vi "Tetra Serial.vi"(0 "COMPORT":refnum<visa-resource-name>="COM4", 1 "Delay Time (ms)":dbl=1.0 caption="Delay Time (s)", 7 "ClearErrorIn(t)":bool=TRUE, 9 "Timeout(s)":dbl=10.0 format="%#_13g", 11 "error in (no error)":errorcluster, 12 "Command":string, 13 "Open Ser(t)":bool, 14 "Close Ser(t)":bool) -> (2 "Success":bool=TRUE, 3 "output":string="adcframe\r\nADC0 Frame: 0x3000800600800655\r\nADC1 Frame: 0x31FF2FF2FF2FF214\r\nADC2 Frame: 0x32FF6FF6FF7FF651\r\nADC3 Frame: 0x33FF1FF0FF3FF033\r\n>", 4 "comport":refnum<visa-resource-name>="COM4", 8 "Timeout":bool caption="Time has Elapsed", 15 "error out":errorcluster)   [LabVIEW 2018]
doc: "This example performs writes and reads on a serial port, as directed by the user. You can press the Write and Read buttons, and change the Read Count, while the example is running.\n\nThe parameters set for the serial port must match the parameters of the connected instrument or device. In this example, the Read Count parameter specifies the number of bytes that the serial port reads. If there were more bytes at the port than the specified number, those bytes would not be read. If there were less bytes at the port than the specified number, you would receive a timeout error.\n\nThis example expands upon the flow control options for XON and XOFF, allowing the user to choose those control characters. Also, the user can enable or disable a termination character. Some devices require a termination character in order to identify the end of command strings. Some devices send a termination character to signify the end of data to be read. This example shows how you can end the Read operation once a termination character is detected in the buffer and/or append a termination character at the end of the Write data."
uses:
  Program Files (x86)/National Instruments/LabVIEW 2018/examples/Instrument IO/Serial/support/Serial - Settings.ctl
  Program Files (x86)/National Instruments/LabVIEW 2018/examples/Instrument IO/Serial/support/Serial - XON-XOFF Characters.ctl
  Program Files (x86)/National Instruments/LabVIEW 2018/examples/Instrument IO/Serial/support/Serial - ASCII Characters.ctl
  <vilib>/Instr/_visa.llb/VISA Flush IO Buffer Mask.ctl
  <vilib>/Utility/error.llb/DialogType.ctl
  Tetra_Globals.vi
  <vilib>/Instr/_visa.llb/VISA Configure Serial Port (Instr).vi
panel:
  out "before substring":string
  out "VI Name":string="Tetra Serial.vi"
  out "x > y?":bool
  in  "set size (in Mbytes)":i64=60
  out "size (in bytes)":i64=140690
  out "file or folder exists?":bool=TRUE
  out "NaN/Path/Refnum?":bool
  out "record id":string="02222023100252"
  in  "Tab Control":enum32{"Page 1", "Page 2"}(tab)
  in  "-ssid":string="123"
  out "Error":bool=TRUE
  out "Elapsed Time (s)":dbl=2.479999966453761e-05
  out "Time(s)":dbl=0.03430839999964519
  in  "x":bool
  in  "LogCapturestoFile":bool
  out "LogFilePath":string="C:\\RageATE Results\\Serial Logs\\02222023100252.txt"
  in  "Read Count":u32=1
  out "return count":u32=8
  out "Numeric Control":i32=138
  in  "Max Lines to Read":i32=1000
  in  "Serial Settings":T1={"baud rate"=115200, "data bits"=8, "parity"=enum."None", "stop bits"=10, "flow control"=0} {"flow control" items=["None"=0, "XON/XOFF"=1, "RTS/CTS"=2, "DTR/DSR"=4]; "stop bits" items=["1.0"=10, "1.5"=15, "2.0"=20]; "data bits" min=5 max=8 step=1; "baud rate" items=["75"=75, "110"=110, "134"=134, "150"=150, "300"=300, "600"=600, "1200"=1200, "1800"=1800, "2400"=2400, "4800"=4800, "7200"=7200, "9600"=9600, "14400"=14400, "19200"=19200, "28800"=28800, "38400"=38400, "56000"=56000, "57600"=57600, "115200"=115200, "128000"=128000, "230400"=230400]}
  in  "XON/XOFF Characters":T2={"XON"=enum."DC1", "XOFF"=enum."DC3"}
  in  "Termination Character":u8=10 format="%.0x"
  out "refnum out":refnum<file>
  out "Start(s)":dbl=8979.5775258 format="%_19f"
  out "log":string="id: 02222023100252 date: 22/02/23  12:18:52.6692  OpenSer: FALSE CloseSer: FALSE  success: TRUE  timeout: FALSE  comport: COM4  cmd: adcframe  return: adcframe;ADC0 Frame: 0x3000800600800655;ADC1 Frame: 0x31FF2FF2FF2FF214;ADC2 Frame: 0x32FF6FF6FF7FF651;ADC3 Frame: 0x33FF1FF0FF3FF033;>"
  # "0xA is equivalent to a '\\n' character, which is a line feed."
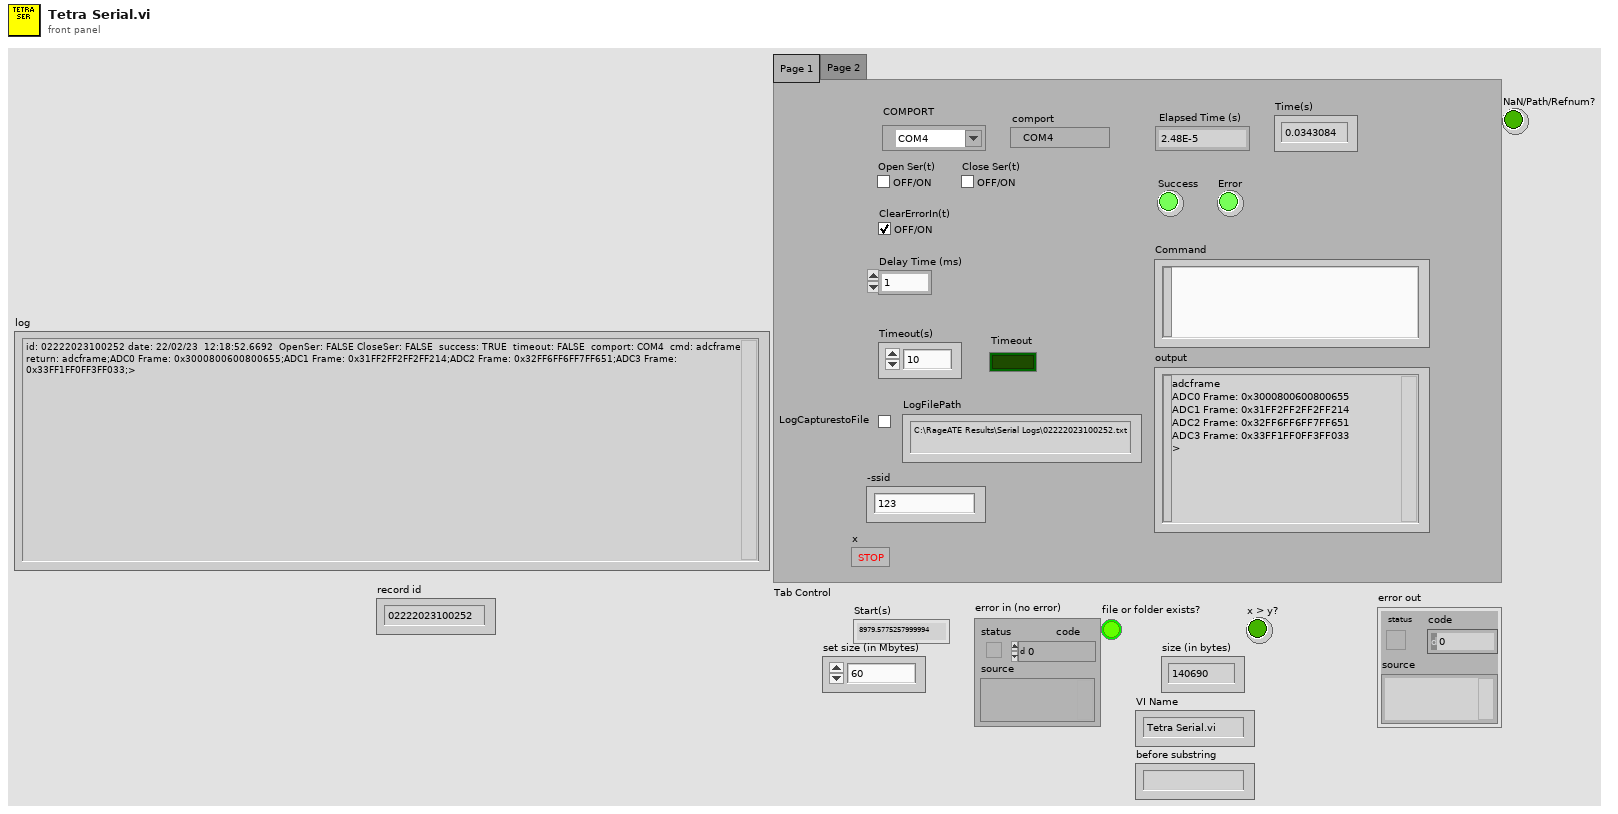
[diagram p1: front panel]
types:
  T1 = typedef "Serial - Settings.ctl" = cluster{"baud rate":u32, "data bits":u16, "parity":enum16{"None", "Odd", "Even", "Mark", "Space"}, "stop bits":u16, "flow control":u16}
  T2 = typedef "Serial - XON-XOFF Characters.ctl" = cluster{"XON":T3, "XOFF":T3}
  T3 = typedef "Serial - ASCII Characters.ctl" = enum16{"NUL", "SOH", "STX", "ETX", "EOT", "ENQ", "ACK", "BEL", "BS", "HT", "LF", "VT", "FF", "CR", "SO", "SI", "DLE", "DC1", "DC2", "DC3", "DC4", "NAK", "SYN", "ETB", "CAN", "EM", "SUB", "ESC", "FS", "GS", "RS", "US", "SP", "!", "\"", "#", "$", "%", "&", "'", "(", ")", "*", "+", ",", "- (-)", ".", "/", "0", "1", "2", "3", "4", "5", "6", "7", "8", "9", ":", ";", "<", "=", ">", "?", "@", "A", "B", "C", "D", "E", "F", "G", "H", "I", "J", "K", "L", "M", "N", "O", "P", "Q", "R", "S", "T", "U", "V", "W", "X", "Y", "Z", "[", "\\", "]", "^", "_", "`", "a", "b", "c", "d", "e", "f", "g", "h", "i", "j", "k", "l", "m", "n", "o", "p", "q", "r", "s", "t", "u", "v", "w", "x", "y", "z", "{", "|", "}", "~"}
  T4 = enum16{"open", "replace", "create", "open or create", "replace or create", "replace or create with confirmation"}
  T5 = typedef "VISA Flush IO Buffer Mask.ctl" = u16
  T6 = typedef "DialogType.ctl" = u16
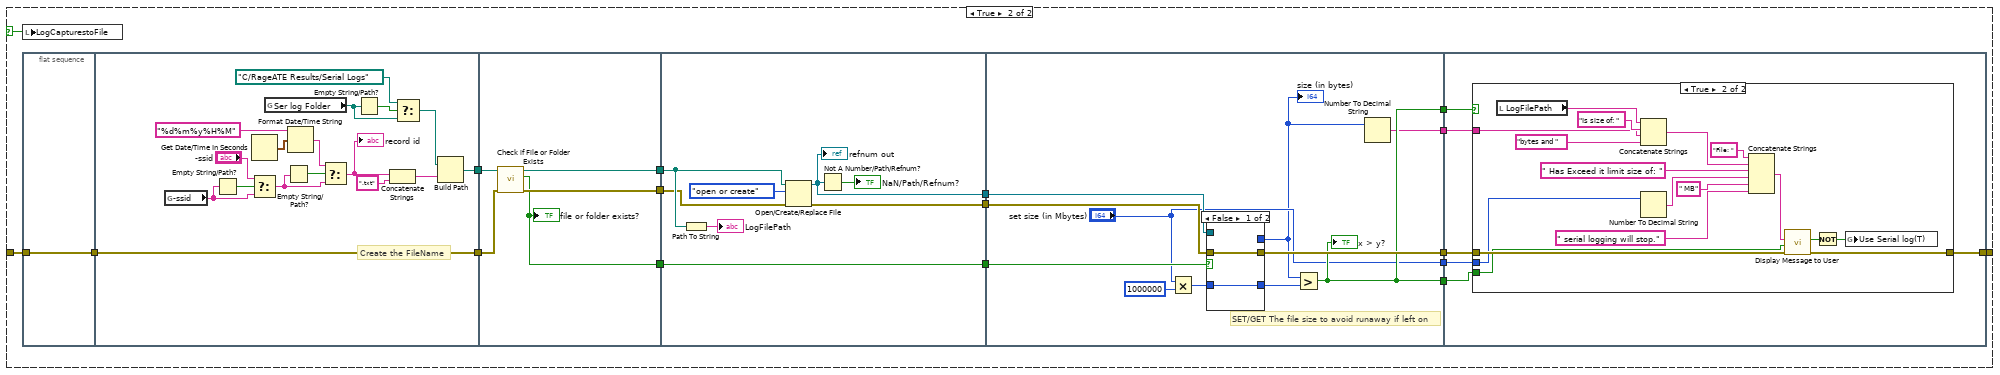
[diagram p2: hidden frame]
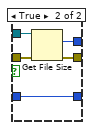
[diagram p3: hidden frame]
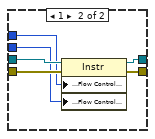
[diagram p8: hidden frame]
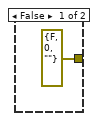
[diagram p9: hidden frame]
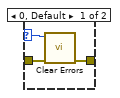
[diagram p10: hidden frame]
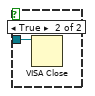
[diagram p12: hidden frame]
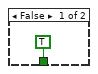
[diagram p14: hidden frame]
diagram:
  n1 = for {
    N: 1 -> [_]
    tunnel: [w5] -> w2
    stop <- w3 stop-if-true
    n2 = flat-sequence {
      tunnel: ["COMPORT"] -> w13
      tunnel: [w17] -> w12
      tunnel: [w118] -> w9
      tunnel: [w117] -> w10
      tunnel: w13 -> [w120]
      tunnel: w12 -> [w119]
      tunnel: [w115] -> w11
      tunnel: [w356] -> w8
      tunnel: [w355] -> w7
      tunnel: w11 -> [w353]
      tunnel: w10 -> [w356]
      tunnel: w9 -> [w355]
      tunnel: [w353] -> w6
      tunnel: w8 -> [_]
      tunnel: w7 -> [w359]
      tunnel: w6 -> [w360]
      tunnel: [w358] -> w4
      tunnel: [w386] -> w5
      tunnel: w4 -> [w386]
      tunnel: [w384] -> w3
      frame #0 {
        n3 = property class="VI"() -> ("Name"=→"VI Name":string)  [unwired: 2 in, 2 out]
        n4 = call <vilib>:"High Resolution Relative Seconds.vi"() -> ("relative seconds"=→"Start(s)":dbl)
        n5 = local write "output"("") -> ()
        n6 = global read "Tetra_Globals.vi" "Use Serial log(T)"() -> (w19:bool)
        n7 = local write "x"(FALSE ("x")) -> ()
        n8 = Or(x="LogCapturestoFile", y=w19) -> (x .or. y?=w20:bool)
        n9 = case shown="False" w20 {
          selector: w20 -> [_ w41]
          tunnel: "error in (no error)" -> [w24 w37]
          tunnel: [w24 w29] -> w17
          frame False {
          }
          frame True {
            n10 = local write "LogCapturestoFile"(w41) -> ()
            n11 = flat-sequence {
              tunnel: w37 -> [w42]
              tunnel: [w42] -> w26
              tunnel: [w45] -> w40
              tunnel: [w43] -> w36
              tunnel: w26 -> [w43]
              tunnel: w40 -> [w62]
              tunnel: [w64] -> w39
              tunnel: [w63] -> w38
              tunnel: w36 -> [w61]
              tunnel: [w60] -> w33
              tunnel: w39 -> [w69]
              tunnel: w38 -> [w70]
              tunnel: [w67] -> w35
              tunnel: [w66] -> w34
              tunnel: w33 -> [w65]
              tunnel: [w65] -> w32
              tunnel: w35 -> [w83]
              tunnel: w34 -> [w82]
              tunnel: w32 -> [w81]
              tunnel: ["set size (in Mbytes)"] -> w31
              tunnel: [w80] -> w30
              tunnel: [w79] -> w28
              tunnel: [w79] -> w27
              tunnel: [w74] -> w25
              tunnel: w31 -> [w94]
              tunnel: w30 -> [w96]
              tunnel: [w95] -> w29
              tunnel: w28 -> [w93]
              tunnel: w27 -> [w92]
              tunnel: w25 -> [w91]
              frame #0 {
              }
              frame #1 {
                # "Create the FileName"
                n12 = global read "Tetra_Globals.vi" "-ssid"() -> (w51:string)
                n13 = Empty String/Path?(string/path=w51) -> (empty?=w52:bool)
                n14 = Get Date/Time In Seconds() -> (seconds since 1Jan1904=w58:timestamp)
                n15 = Select(t="-ssid", s=w52, f=w51) -> (s? t:f=w49:string)
                n16 = global read "Tetra_Globals.vi" "Ser log Folder"() -> (w48:path)
                n17 = Empty String/Path?(string/path=w49) -> (empty?=w59:bool)
                n18 = Format Date/Time String(time format string (%c)="%d%m%y%H%M", seconds (now)=w58) -> (date/time string=w56:string)  [unwired: 1 in]
                n19 = Select(t=w56, s=w59, f=w49) -> (s? t:f=w55:string)
                "record id" <- w55
                n20 = Empty String/Path?(string/path=w48) -> (empty?=w47:bool)
                n21 = Concatenate Strings(w55, ".txt" ("string")) -> (w53:string)
                n22 = Select(t=path "C:/RageATE Results/Serial Logs" ("base path"), s=w47, f=w48) -> (s? t:f=w44:path)
                n23 = Build Path(base path=w44, name or relative path=w53) -> (appended path=w45:path)
              }
              frame #2 {
                n24 = call <vilib>:"Check if File or Folder Exists.vi"("error in (no error)"=w61, "path"=w62) -> ("error out"=w64:errorcluster, "file or folder exists?"=w60:bool, "dup path"=w63:path)  [unwired: 7 in]
                "file or folder exists?" <- w60
              }
              frame #3 {
                n25 = Path To String(path=w70) -> (string=→"LogFilePath":string)
                n26 = Open/Create/Replace File(file path (use dialog)=w70, error in=w69, operation (0:open)=T4."open or create") -> (refnum out=w66:refnum<file>, error out=w67:errorcluster)  [unwired: 3 in, 1 out]
                "refnum out" <- w66
                n27 = Not A Number/Path/Refnum?(number/path/refnum=w66) -> (NaN/Path/Refnum?=→"NaN/Path/Refnum?":bool)
              }
              frame #4 {
                # "SET/GET The file size to avoid runaway if left on"
                n28 = Multiply(x="set size (in Mbytes)", y=i64 1000000) -> (x*y=w76:i64)
                n29 = case shown="False" w81 {
                  tunnel: w83 -> [w84 w89]
                  tunnel: w82 -> [_ w90]
                  tunnel: [_ w86] -> w75
                  tunnel: w76 -> [w85 w87]
                  tunnel: [w84 w88] -> w80
                  tunnel: [w85 w87] -> w73
                  frame False {
                  }
                  frame True {
                    n30 = Get File Size(file=w90, error in=w89) -> (size (in bytes)=w86:i64, 0:w88:errorcluster)  [unwired: 1 out]
                  }
                }
                "size (in bytes)" <- w75
                n31 = Greater?(x=w75, y=w73) -> (0:w79:bool)
                "x > y?" <- w79
                n32 = Number To Decimal String(number=w75) -> (decimal integer string=w74:string)  [unwired: 1 in]
              }
              frame #5 {
                n33 = case shown="True" w92 {
                  tunnel: w96 -> [w97 w114]
                  tunnel: [w97 w113] -> w95
                  tunnel: w94 -> [_ w109]
                  tunnel: w93 -> [_ w105]
                  tunnel: w91 -> [_ w99]
                  frame False {
                  }
                  frame True {
                    n34 = local read "LogFilePath"() -> (w111:string)
                    n35 = Concatenate Strings(w111, "Is size of: " ("string"), w99, "bytes and " ("string")) -> (w101:string)
                    n36 = Number To Decimal String(number=w109) -> (decimal integer string=w108:string)  [unwired: 1 in]
                    n37 = Concatenate Strings("File: ", w101, " Has Exceed it limit size of: " ("string"), w108, " MB" ("string"), " serial logging will stop." ("string")) -> (w106:string)
                    n38 = call "Display Message to User"("error in (no error)"=w114, "Enable"=w105, "Message"=w106) -> ("error out"=w113:errorcluster, "OK"=w104:bool)  [unwired: 7 in]
                    n39 = Not(x=w104) -> (.not. x?=w103:bool)
                    n40 = global write "Tetra_Globals.vi" "Use Serial log(T)"(w103) -> ()
                  }
                }
              }
            }
          }
        }
      }
      frame #1 {
        n41 = for {
          N: 1 -> [_]
          tunnel: w120 -> [w147]
          shift-right: [w146] -> w118
          shift-left: w119 -> [w143]
          tunnel: [w131] -> w117
          shift-right: [w122] -> w115
          shift-left: _ -> [_]
          stop <- w129 continue-if-true
          n42 = flat-sequence {
            tunnel: w147 -> [w151]
            tunnel: [w151] -> w145
            tunnel: [w149] -> w144
            tunnel: w143 -> [w150]
            tunnel: w145 -> [w159]
            tunnel: w144 -> [w156]
            tunnel: [w158] -> w142
            tunnel: [w157] -> w141
            tunnel: w142 -> [w203]
            tunnel: w141 -> [w201]
            tunnel: [w200] -> w140
            tunnel: [w199] -> w139
            tunnel: w140 -> [w208]
            tunnel: w139 -> [w209]
            tunnel: [w207] -> w138
            tunnel: [w206] -> w123
            tunnel: [w205] -> w121
            tunnel: w138 -> [w218]
            tunnel: [w217] -> w137
            tunnel: [w216] -> w124
            tunnel: w123 -> [w216]
            tunnel: w121 -> [w215]
            tunnel: w137 -> [w226]
            tunnel: [w225] -> w136
            tunnel: [w224] -> w135
            tunnel: [w223] -> w134
            tunnel: w124 -> [w222]
            tunnel: w136 -> [w292]
            tunnel: w135 -> [w290]
            tunnel: w134 -> [w291]
            tunnel: [w292] -> w133
            tunnel: [w289] -> w132
            tunnel: w133 -> [w299]
            tunnel: w132 -> [w301]
            tunnel: [w297] -> w129
            tunnel: [w298] -> w130
            tunnel: [w297] -> w128
            tunnel: w130 -> [w304]
            tunnel: w128 -> [w303]
            tunnel: [w304] -> w126
            tunnel: [w302] -> w125
            tunnel: [w351] -> w127
            tunnel: [w352] -> w131
            tunnel: w126 -> [w352]
            tunnel: w125 -> [w351]
            tunnel: [w342] -> w122
            frame #0 {
              n43 = case shown="True" "ClearErrorIn(t)" {
                tunnel: w150 -> [w152 w154]
                tunnel: [w152 w153] -> w149
                frame False {
                }
                frame True {
                  n44 = call <vilib>:"Clear Errors.vi"("error in (no error)"=w154) -> ("error out"=w153:errorcluster)  [unwired: 5 in, 1 out]
                }
              }
            }
            frame #1 {
              n45 = case shown="True" "Open Ser(t)" {
                tunnel: w159 -> [w161 w162]
                tunnel: [w160 w168] -> w158
                tunnel: [w161 w164] -> w157
                tunnel: w156 -> [w160 w163]
                frame False {
                }
                frame True {
                  w166 = TRUE  # End Write on Termination Character?
                  w173 = TRUE  # End Read on Termination Character?
                  n46 = Unbundle By Name("Serial Settings") -> ("baud rate"=w175:u32, "data bits"=w176:u16, "parity"=w177:enum16{"None", "Odd", "Even", "Mark", "Space"}, "stop bits"=w178:u16, "flow control"=w172:u16)
                  n47 = Unbundle By Name("XON/XOFF Characters") -> ("XON"=w171:T3, "XOFF"=w170:T3)
                  n48 = call-poly "VISA Configure Serial Port"("VISA resource name"=w162, "termination char\n(0xA = '\\n' = LF)"="Termination Character", "Enable Termination\nChar (T)"=w173, "baud rate (9600)"=w175, "data bits (8)"=w176, "parity (0:none)"=w177, "error in (no error)"=w163, "stop bits (10: 1 bit)"=w178, "flow control (0:none)"=w172) -> ("VISA resource name out"=w179:refnum<visa-resource-name>, "error out"=w180:errorcluster)  [unwired: 1 in, 4 out]
                  n49 = case shown="Default" w172 {
                    tunnel: [w191 w198] -> w169
                    tunnel: [w192 w197] -> w167
                    tunnel: w180 -> [w191 w196]
                    tunnel: w179 -> [w192 w195]
                    tunnel: w171 -> [_ w194]
                    tunnel: w170 -> [_ w193]
                    frame Default {
                    }
                    frame 1 {
                      n50 = property class="Instr"(reference=w195, error in=w196, "Serial Settings:Flow Control XON Character"=w194, "Serial Settings:Flow Control XOFF Character"=w193) -> (reference out=w197:refnum<visa-resource-name>, error out=w198:errorcluster)
                    }
                  }
                  n51 = case shown="True" w166 {
                    tunnel: w167 -> [w182 w190]
                    tunnel: w169 -> [w183 w189]
                    tunnel: [w182 w188] -> w164
                    tunnel: [w183 w187] -> w168
                    tunnel: "Termination Character" -> [_ w185]
                    frame False {
                    }
                    frame True {
                      w186 = u16 2 items=["None", "LastBit", "TermChar", "Break"] ("Serial Settings:Serial End Mode for Writes")
                      n52 = property class="Instr"(reference=w190, error in=w189, "Serial Settings:End Mode for Writes"=w186, "Message Based Settings:Send End Enable"=TRUE, "Message Based Settings:Termination Character"=w185) -> (reference out=w188:refnum<visa-resource-name>, error out=w187:errorcluster)
                    }
                  }
                }
              }
            }
            frame #2 {
              w202 = T5 64 items=["Flush Receive Buffer"=16, "Write Transmit Buffer to Device"=32, "Flush Receive Buffer (No I/O)"=64, "Flush Transmit Buffer"=128] ("Mask")
              n53 = VISA Flush I/O Buffer(VISA resource name=w201, mask (16)=w202, error in (no error)=w203) -> (VISA resource name out=w199:refnum<visa-resource-name>, error out=w200:errorcluster)
            }
            frame #3 {
              n54 = VISA Write(VISA resource name=w209, write buffer="Command", error in (no error)=w208) -> (VISA resource name out=w206:refnum<visa-resource-name>, return count=w205:u32, error out=w207:errorcluster)
              "return count" <- w205
            }
            frame #4 {
              n55 = Greater?(x=w215, y=u32 1) -> (0:w213:bool)
              n56 = Select(t=5.0 ("x"), s=w213, f=1.0 ("x")) -> (s? t:f=w210:dbl)
              n57 = Divide(x=w210, y=1000.0) -> (x/y=w220:dbl)
              n58 = call "Time Delay"("error in (no error)"=w218, "Delay Time (s)"=w220) -> ("error out"=w217:errorcluster)  [unwired: 9 in]
            }
            frame #5 {
              # "ERR:"
              # "Unknown command"
              n59 = while {
                shift-right: [w242] -> w225
                shift-left: w222 -> [w240]
                tunnel: [w239] -> w224
                tunnel: w226 -> [w241]
                tunnel: [w238] -> w223
                border: "" -> [_]
                i -> [w230]
                stop <- w231 stop-if-true
                # "Serial Write and Read Loop"
                n60 = flat-sequence {
                  tunnel: w240 -> [w245]
                  tunnel: w241 -> [w244]
                  tunnel: [w244] -> w233
                  tunnel: [w245] -> w232
                  tunnel: [w243] -> w229
                  tunnel: w230 -> [w266]
                  tunnel: [w254] -> w237
                  tunnel: [w267] -> w236
                  tunnel: [w261] -> w235
                  tunnel: [w260] -> w234
                  tunnel: w233 -> [w263]
                  tunnel: w232 -> [w262]
                  tunnel: w229 -> [w247]
                  tunnel: [w247] -> w228
                  tunnel: [w280] -> w238
                  tunnel: [w274] -> w239
                  tunnel: [w281] -> w242
                  tunnel: w236 -> [w281]
                  tunnel: w235 -> [w273]
                  tunnel: w234 -> [w280]
                  tunnel: w228 -> [w277]
                  tunnel: [w272] -> w227
                  frame #0 {
                    n61 = call <vilib>:"High Resolution Relative Seconds.vi"() -> ("relative seconds"=w243:dbl)
                  }
                  frame #1 {
                    w256 = string[] ["Unknown command", "ERR:", "ERR: No PFD link (-40)"]  # list of bad readback
                    n62 = Equal?(x="Max Lines to Read", y=w266) -> (x = y?=w264:bool)
                    n63 = VISA Read(VISA resource name=w262, byte count="Read Count", error in (no error)=w263) -> (VISA resource name out=w267:refnum<visa-resource-name>, read buffer=w250:string, error out=w261:errorcluster)  [unwired: 1 out]
                    n64 = Unbundle By Name(w261) -> ("code"=w260:i32)
                    n65 = feedback #1() -> (w251:string)
                    n66 = call <vilib>:"Trim Whitespace.vi"("string"=w250) -> ("trimmed string"=w249:string)  [unwired: 1 in]
                    n67 = Concatenate Strings(w251, w250) -> (w257:string)
                    "output" <- w257
                    n68 = feedback-in #1(w257) -> ()
                    n69 = for {
                      tunnel: w257 -> [w271]
                      tunnel: w256 -> [w270] mode=indexing
                      tunnel: [w268] -> w255
                      tunnel: [w269] -> w246 if=w268
                      n70 = Match Pattern(string=w271, regular expression=w270) -> (match substring=w269:string)  [unwired: 1 in, 3 out]
                      n71 = Equal?(x=w269, y=w270) -> (x = y?=w268:bool)
                    }
                    "Error" <- w255
                    "before substring" <- w246
                    n72 = Or(x="x", y=w264) -> (x .or. y?=w259:bool)
                    n73 = Equal?(x=w249, y=">" ("true string")) -> (x = y?=w253:bool)
                    "Success" <- w253
                    n74 = Or(x=w253, y=w259) -> (x .or. y?=w254:bool)
                    "Numeric Control" <- w266
                  }
                  frame #2 {
                    n75 = call <vilib>:"High Resolution Relative Seconds.vi"() -> ("relative seconds"=w278:dbl)
                    n76 = Subtract(x=w278, y=w277) -> (x-y=w276:dbl)
                    "Elapsed Time (s)" <- w276
                    n77 = Greater Or Equal?(x=w276, y="Timeout(s)") -> (x >= y?=w272:bool)
                    "Timeout" <- w272
                    n78 = case shown="True" w272 {
                      tunnel: [errorcluster {"status"=FALSE, "code"=0, "source"=""} ("error out") w288] -> w279
                      frame False {
                      }
                      frame True {
                        w287 = T6 2 items=["no dialog", "OK message", "continue or stop message", "OK message + warnings", "continue/stop + warnings"] ("type of dialog (OK msg:1)")
                        n79 = local read "VI Name"() -> (w284:string)
                        n80 = Concatenate Strings("Operation Timeout In : ", w284) -> (w283:string)
                        n81 = call <vilib>:"General Error Handler.vi"("[error code] (0)"=0, "[error source] (\" \")"=w283, "type of dialog (OK msg:1)"=w287) -> ("error out"=w288:errorcluster)  [unwired: 8 in, 4 out]
                      }
                    }
                    n82 = Merge Errors(w273, w279) -> (w274:errorcluster)
                  }
                }
                n83 = Equal To 0?(x=w230) -> ()  [unwired: 1 out]
                n84 = Or(x=w227, y=w237) -> (x .or. y?=w231:bool)
              }
            }
            frame #6 {
              # "Only clear erro from overflow"
              n85 = case shown="-1073807339" w291 {
                selector: w291 -> [w293 _]
                tunnel: w290 -> [w295 w296]
                tunnel: [w294 w296] -> w289
                frame 0, Default {
                  n86 = call <vilib>:"Clear Errors.vi"("error in (no error)"=w295, "specific error code to clear (0: all)"=w293) -> ("error out"=w294:errorcluster)  [unwired: 4 in, 1 out]
                }
                frame -1073807339 {
                }
              }
            }
            frame #7 {
              w300 = T5 16 items=["Flush Receive Buffer"=16, "Write Transmit Buffer to Device"=32, "Flush Receive Buffer (No I/O)"=64, "Flush Transmit Buffer"=128] ("Mask")
              n87 = VISA Flush I/O Buffer(VISA resource name=w299, mask (16)=w300, error in (no error)=w301) -> (VISA resource name out=w298:refnum<visa-resource-name>, error out=w297:errorcluster)
            }
            frame #8 {
              n88 = case shown="Error" w303 {
                selector: w303 -> [w305 w306]
                tunnel: [w305 w306] -> w302
                frame No Error {
                }
                frame Error {
                  n89 = local write "Open Ser(t)"(TRUE ("Open Ser(t)")) -> ()
                }
              }
            }
            frame #9 {
              w325 = ";"
              w323 = TRUE ("replace all? (F)")
              n90 = local read "output"() -> (w329:string)
              n91 = Search and Replace String(replace all?=w323, case sensitive?=w323, input string=w329, search string="\\n\\r", replace string=w325) -> (result string=w327:string)  [unwired: 3 in, 3 out]
              n92 = Divide(x="Delay Time (ms)", y=1000.0) -> (x/y=w310:dbl)
              n93 = local read "Timeout"() -> (w338:bool)
              n94 = call "Time Delay2"("Delay Time (s)"=w310) -> ()  [unwired: 10 in, 1 out]
              n95 = Search and Replace String(replace all?=w323, case sensitive?=w323, input string=w327, search string="\\r\\n", replace string=w325) -> (result string=w324:string)  [unwired: 3 in, 3 out]
              n96 = local read "Open Ser(t)"() -> (w335:bool)
              n97 = local read "Close Ser(t)"() -> (w334:bool)
              n98 = local read "Command"() -> (w321:string)
              n99 = local read "record id"() -> (w315:string)
              n100 = Select(t=" timed out  ", s=w338, f=w324) -> (s? t:f=w318:string)
              n101 = local read "COMPORT"() -> (w312:refnum<visa-resource-name>)
              n102 = local read "Timeout"() -> (w340:bool)
              n103 = local read "Success"() -> (w345:bool)
              n104 = Format Into String(initial string=" OpenSer: ", w335) -> (resulting string=w332:string)  [unwired: 2 in, 1 out]
              n105 = Format Into String(initial string=" CloseSer: ", w334) -> (resulting string=w331:string)  [unwired: 2 in, 1 out]
              n106 = Get Date/Time In Seconds() -> (seconds since 1Jan1904=w350:timestamp)
              n107 = Concatenate Strings("id: " ("string"), w315) -> (w314:string)
              n108 = Format Date/Time String(time format string (%c)="%d/%m/%y  %H:%M:%S%4u ", seconds (now)=w350) -> (date/time string=w348:string)  [unwired: 1 in]
              n109 = Concatenate Strings(w332, w331) -> (w330:string)
              n110 = Format Into String(initial string="  success: ", w345) -> (resulting string=w344:string)  [unwired: 2 in, 1 out]
              n111 = Format Into String(initial string="  timeout: ", w340) -> (resulting string=w339:string)  [unwired: 2 in, 1 out]
              n112 = Concatenate Strings("  comport: " ("string"), w312) -> (w311:string)
              n113 = Concatenate Strings("  cmd: " ("string"), w321) -> (w320:string)
              n114 = Concatenate Strings("  return: " ("string"), w318) -> (w317:string)
              n115 = call <vilib>:"Space Constant.vi"() -> ("String"=w346:string)
              n116 = Concatenate Strings(w314, w346, "date: " ("string"), w348, w330, w344, w339, w311, w320, w317) -> (w342:string)
              "log" <- w342
            }
          }
          n117 = Merge Errors(w127) -> (w146:errorcluster)
        }
      }
      frame #2 {
        n118 = local read "Close Ser(t)"() -> (w354:bool)
        n119 = case shown="False" w354 {
          tunnel: w356 -> [_ w357]
          frame False {
          }
          frame True {
            n120 = VISA Close(VISA resource name=w357) -> ()  [unwired: 1 in, 1 out]
          }
        }
        "comport" <- w356
      }
      frame #3 {
        n121 = local read "Start(s)"() -> (w363:dbl)
        n122 = local read "LogCapturestoFile"() -> (w361:bool)
        n123 = call <vilib>:"High Resolution Relative Seconds.vi"() -> ("relative seconds"=w362:dbl)
        n124 = Subtract(x=w362, y=w363) -> (x-y=w364:dbl)
        "Time(s)" <- w364
        n125 = case shown="True" w361 {
          tunnel: w360 -> [_ w379]
          tunnel: w364 -> [_ w369]
          tunnel: w359 -> [w365 w367]
          tunnel: [w365 w366] -> w358
          frame False {
          }
          frame True {
            n126 = local read "refnum out"() -> (w383:refnum<file>)
            n127 = local read "file or folder exists?"() -> (w374:bool)
            n128 = Number To Fractional String(number=w369) -> (F-format string=w368:string)  [unwired: 3 in]
            n129 = Concatenate Strings(w379, " elapsed time: " ("string"), w368) -> (w371:string)
            n130 = Get File Position(4:w367, 7:w383) -> (0:w377:errorcluster, 3:w382:refnum<file>)  [unwired: 1 out]
            n131 = Select(t="\r\n", s=w374, f="") -> (s? t:f=w375:string)
            n132 = Concatenate Strings(w375, w371) -> (w376:string)
            n133 = Set File Position(refnum=w382, from (0:start)=enum16{"start", "end", "current"}."end", error in=w377) -> (refnum out=w380:refnum<file>, error out=w378:errorcluster)  [unwired: 1 in]
            n134 = Write to Text File(file (use dialog)=w380, text=w376, error in=w378) -> (error out=w366:errorcluster)  [unwired: 1 in, 2 out]
          }
        }
      }
      frame #4 {
        # "There is a problem with the USB connection."
        n135 = local read "Error"() -> (w385:bool)
        n136 = case shown="True" w385 {
          tunnel: [TRUE ("OK") w390] -> w384
          frame False {
          }
          frame True {
            n137 = local write "Success"(FALSE ("Success")) -> ()
            n138 = call "Display Message to User2"() -> ("OK"=w390:bool)  [unwired: 10 in, 1 out]
            n139 = local write "output"("There is a problem with the USB connection. ") -> ()
          }
        }
      }
    }
  }
  "error out" <- w2
